vi "RT Driver_Global.vi"() -> ()   [LabVIEW 2013, in "SNTP Light Custom Device Engine.lvlib"]
uses:
  SNTP Light Custom Device Engine.lvlib
panel:
  out "session out":refnum<k21> caption="Systen Configuration session out"
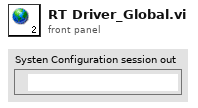
[diagram p1: front panel]
diagram:
